vi "Sprite_RunLengthEncode.vi"(11 "64 Color Images (Concatenated)":fxp<+,6,6>[](array[numeric])) -> (2 "Indexes":u32[](array[numeric]), 3 "RLE Images":fxp<+,12,12>[](array[numeric]))   [LabVIEW 2020]
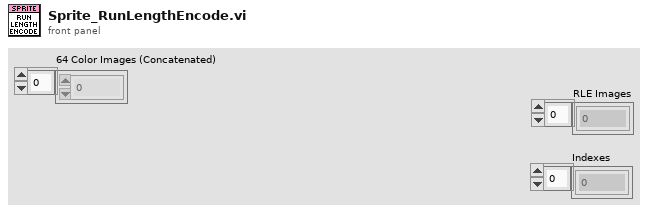
[diagram p1: front panel]
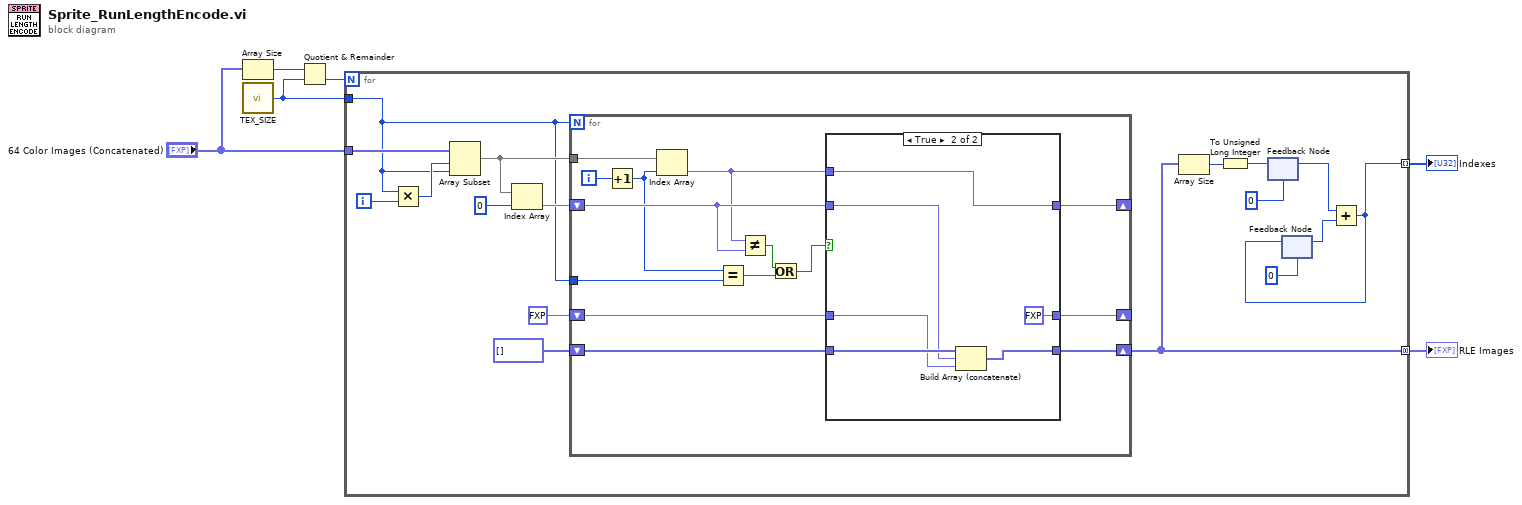
[diagram p0: block diagram]
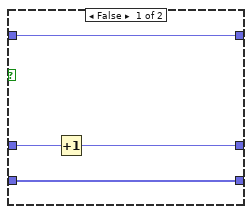
[diagram p2: hidden frame]
diagram:
  n1 = Array Size(array="64 Color Images (Concatenated)") -> (size(s)=w6:i32)
  n2 = call "TEX_SIZE.vi"() -> ("TEX_SIZE"=w4:u32)
  n3 = Quotient & Remainder(x=w6, y=w4) -> (floor(x/y)=w1:u32)  [unwired: 1 out]
  n4 = for {
    N: w1 -> [_]
    tunnel: "64 Color Images (Concatenated)" -> [w23]
    tunnel: w4 -> [w7]
    tunnel: [w9] -> w3 mode=indexing
    tunnel: [w14] -> w2 mode=concatenating
    i -> [w22]
    n5 = Multiply(x=w7, y=w22) -> (x*y=w21:u32)
    n6 = Array Subset(array=w23, index=w21, length=w7) -> (w18:fxp<+,6,6>[])
    n7 = Index Array(array=w18, index=0) -> (element=w19:fxp<+,6,6>)
    n8 = for {
      N: w7 -> [_]
      shift-right: [w31] -> _
      shift-left: w19 -> [w34]
      tunnel: w18 -> [w37]
      shift-right: [w35] -> _
      shift-left: fxp<+,12,12> 1.0 ("index") -> [w36]
      shift-right: [w30] -> w14
      shift-left: fxp<+,12,12>[] [] -> [w33]
      tunnel: w7 -> [w28]
      i -> [w29]
      n9 = Increment(x=w29) -> (x+1=w27:i32)
      n10 = Index Array(array=w37, index=w27) -> (element=w32:fxp<+,6,6>)
      n11 = Equal?(x=w27, y=w28) -> (x = y?=w26:bool)
      n12 = Not Equal?(x=w32, y=w34) -> (x != y?=w25:bool)
      n13 = Or(x=w25, y=w26) -> (x .or. y?=w24:bool)
      n14 = case shown="True" w24 {
        tunnel: w36 -> [w41 w43]
        tunnel: [w40 fxp<+,12,12> 1.0] -> w35
        tunnel: w34 -> [w38 w45]
        tunnel: w33 -> [w39 w46]
        tunnel: w32 -> [_ w44]
        tunnel: [w38 w44] -> w31
        tunnel: [w39 w42] -> w30
        frame False {
          n15 = Increment(x=w41) -> (x+1=w40:fxp<+,12,12>)
        }
        frame True {
          n16 = Build Array (concatenate)(w46, w45, w43) -> (w42:fxp<+,12,12>[])
        }
      }
    }
    n17 = Array Size(array=w14) -> (size(s)=w12:i32)
    n18 = To Unsigned Long Integer(number=w12) -> (unsigned 32bit integer=w13:u32)
    n19 = feedback #1(u32 0) -> (w11:u32)
    n20 = feedback-in #1(w13) -> ()
    n21 = feedback #2(u32 0) -> (w10:u32)
    n22 = Add(x=w11, y=w10) -> (x+y=w9:u32)
    n23 = feedback-in #2(w9) -> ()
  }
  "Indexes" <- w3
  "RLE Images" <- w2
